vi "StringToArray.vi"(1 "spreadsheet string":string) -> (0 "array":string[](array[string]))   [LabVIEW 2016]
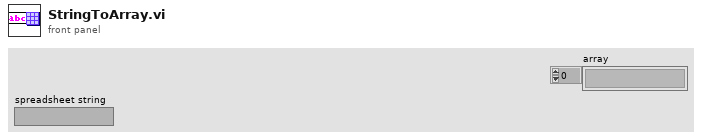
[diagram p1: front panel]
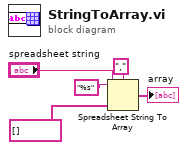
[diagram p0: block diagram]
diagram:
  n1 = Spreadsheet String To Array(delimiter (Tab)=",", format string="%s", spreadsheet string="spreadsheet string", array type (2D Dbl)=string[] []) -> (array=→"array":string[])
